vi "Move Motors.vi"(8 "Camera Resolution X":i64, 9 "pix/micron":dbl, 10 "XY Mouse Position":string, 11 "Current Motor Position past home (um)":string) -> (5 "Motor XY After Moving":string)   [LabVIEW 2014]
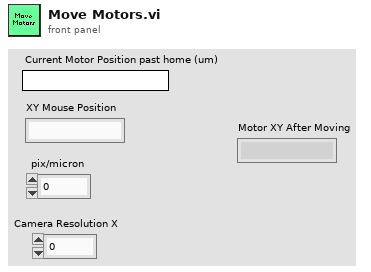
[diagram p1: front panel]
types:
  T1 = enum16{"Default", "Set Statuses", "Set Parameters", "Save Parameter"}
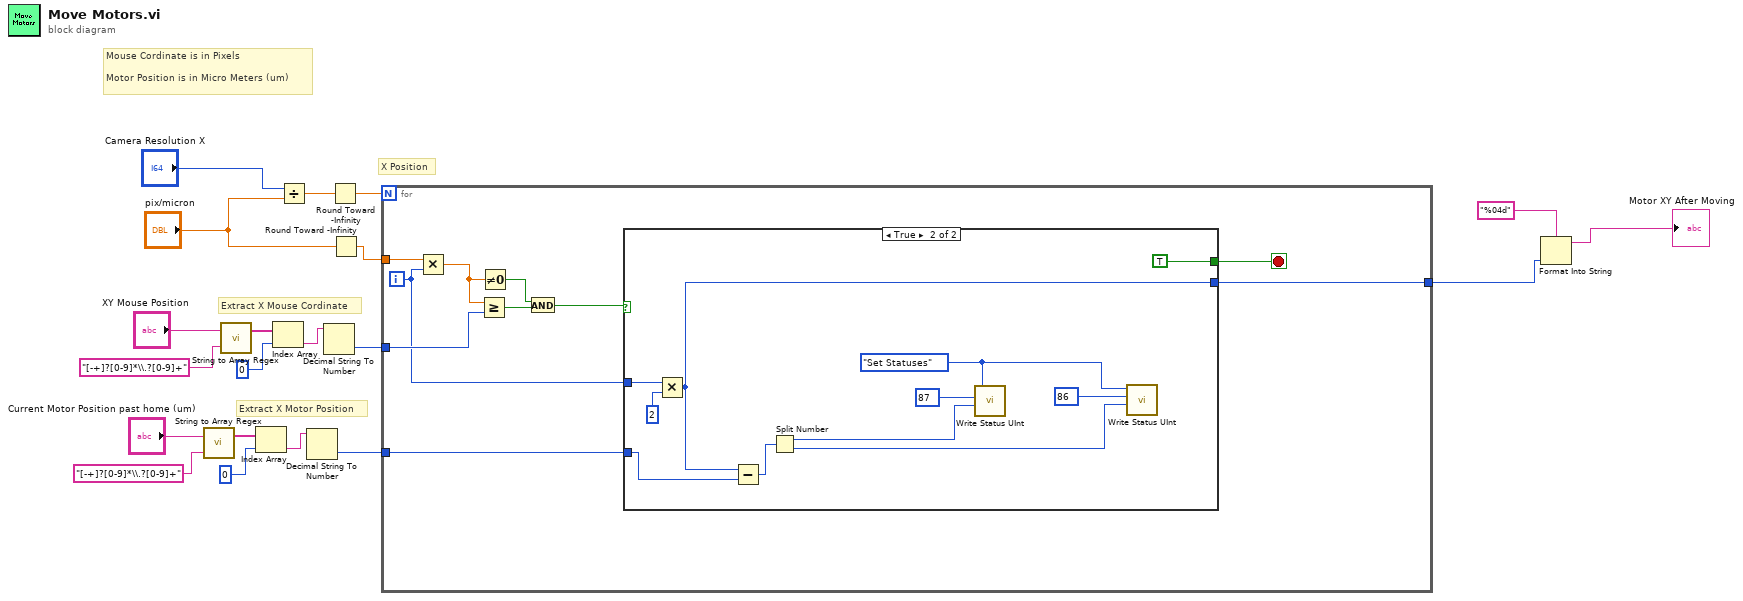
[diagram p0: block diagram]
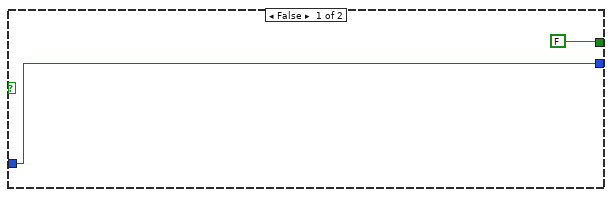
[diagram p2: hidden frame]
diagram:
  # "Mouse Cordinate is in Pixels\n\nMotor Position is in Micro Meters (um)"
  # "Extract X Motor Position"
  # "Extract X Mouse Cordinate"
  # "X Position"
  n1 = call "String to Array Regex.vi"("Regex"="[-+]?[0-9]*\\.?[0-9]+", "Message"="Current Motor Position past home (um)") -> ("String to Array"=w11:string[])  [unwired: 1 in]
  n2 = call "String to Array Regex.vi"("Regex"="[-+]?[0-9]*\\.?[0-9]+", "Message"="XY Mouse Position") -> ("String to Array"=w15:string[])  [unwired: 1 in]
  n3 = Index Array(array=w11, index=0) -> (element=w9:string)
  n4 = Index Array(array=w15, index=0) -> (element=w12:string)
  n5 = Divide(x="Camera Resolution X", y="pix/micron") -> (x/y=w18:dbl)
  n6 = Decimal String To Number(string=w9) -> (number=w7:i32)  [unwired: 2 in, 1 out]
  n7 = Decimal String To Number(string=w12) -> (number=w13:i32)  [unwired: 2 in, 1 out]
  n8 = Round Toward -Infinity(1:w18) -> (0:w19:dbl)
  n9 = Round Toward -Infinity(1:"pix/micron") -> (0:w4:dbl)
  n10 = for {
    N: w19 -> [_]
    tunnel: w13 -> [w30]
    tunnel: w7 -> [w29]
    tunnel: w4 -> [w23]
    tunnel: [w22] -> w1
    i -> [w21]
    stop <- w24 stop-if-true
    n11 = Multiply(x=w23, y=w21) -> (x*y=w25:dbl)
    n12 = Greater Or Equal?(x=w25, y=w30) -> (x >= y?=w28:bool)
    n13 = Not Equal To 0?(x=w25) -> (x != 0?=w27:bool)
    n14 = And(x=w27, y=w28) -> (x .and. y?=w26:bool)
    n15 = case shown="True" w26 {
      tunnel: w29 -> [_ w34]
      tunnel: [FALSE TRUE] -> w24
      tunnel: [w31 w33] -> w22
      tunnel: w21 -> [w31 w36]
      frame False {
      }
      frame True {
        w42 = T1."Set Statuses" ("Command")
        n16 = Multiply(x=w36, y=2) -> (x*y=w33:i32)
        n17 = Subtract(x=w33, y=w34) -> (x-y=w35:i32)
        n18 = Split Number(x=w35) -> (hi(x)=w40:u16, lo(x)=w39:u16)
        n19 = call "Write Status UInt.vi"("Status Value"=w40, "Status Number"=u16 87 ("Status Value"), "Command"=w42) -> ()  [unwired: 4 in, 1 out]
        n20 = call "Write Status UInt.vi"("Status Value"=w39, "Status Number"=u16 86 ("Status Value"), "Command"=w42) -> ()  [unwired: 4 in, 1 out]
      }
    }
  }
  n21 = Format Into String(format string="%04d", w1) -> (resulting string=→"Motor XY After Moving":string)  [unwired: 2 in, 1 out]
